vi "Input_Instrument_Positions.vi"(1 "Filepath to Save":path) -> (0 "Output string":string)   [LabVIEW 2010]
uses:
  Controls/ok_button.ctl
  Globals/Meas_global.vi
  Globals/Constants_global.vi
  Globals/Trav_pos_global.vi
panel:
  in  "OK":T1
  in  "Instrument positions when the traverse is at its origin":T2(array[cluster])=[{"Name"="", "X"=0.0, "Y"=0.0, "Z"=0.0, "Mounted On"=0}] {"Mounted On" items=["None", "No Traverse", "Tunnel3Traverse"]; "Z" format="%#.2f"; "Y" format="%#.2f"; "X" format="%#.2f"}
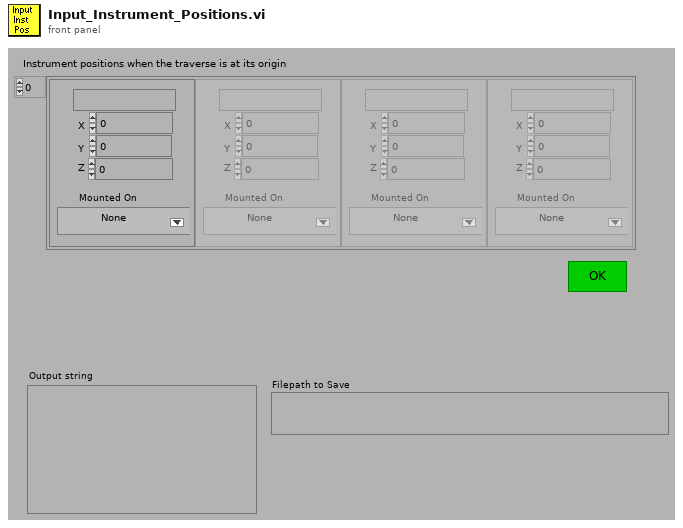
[diagram p1: front panel]
types:
  T1 = typedef "ok_button.ctl" = bool
  T2 = cluster{"Name":string, "X":dbl, "Y":dbl, "Z":dbl, "Mounted On":u16}[]
  T3 = cluster{"Name":string, "X":dbl, "Y":dbl, "Z":dbl}[]
  T4 = cluster{"Name":string, "X":dbl, "Y":dbl, "Z":dbl, "Mounted On":u16}
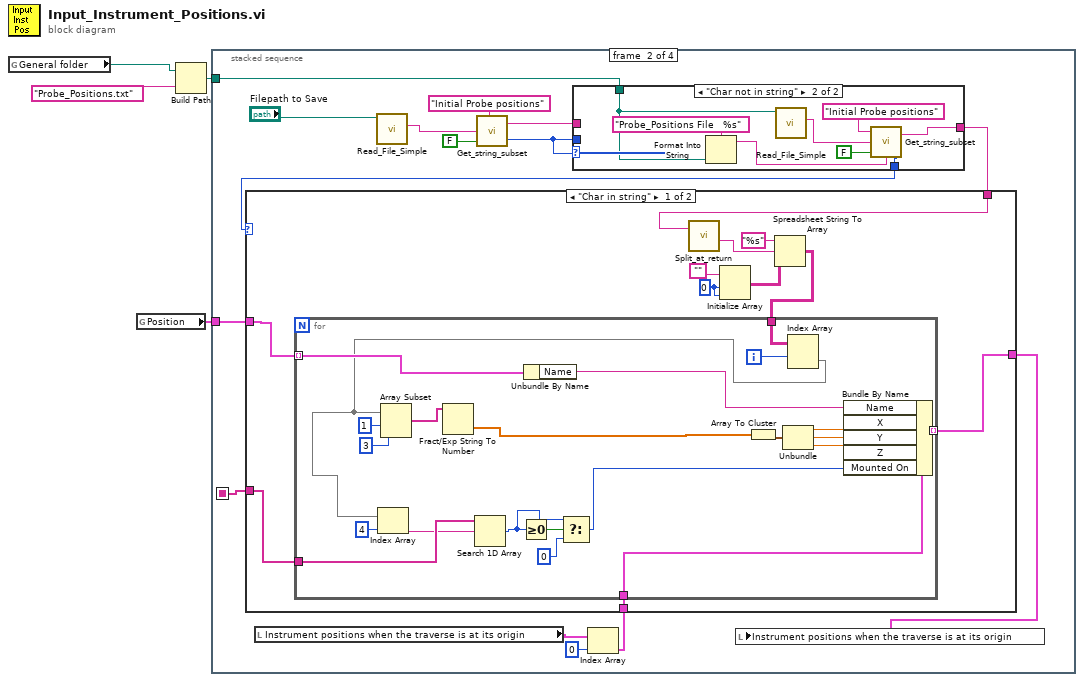
[diagram p0: block diagram]
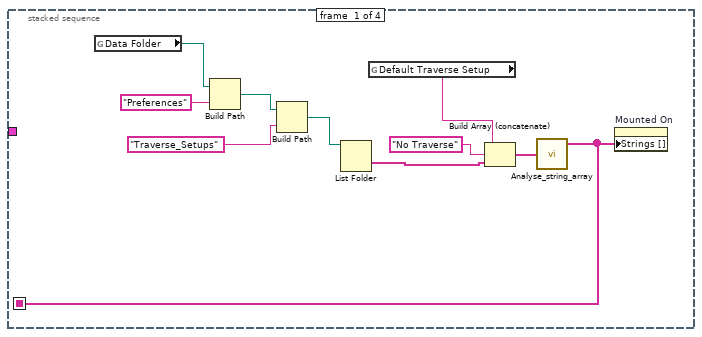
[diagram p2: hidden frame]
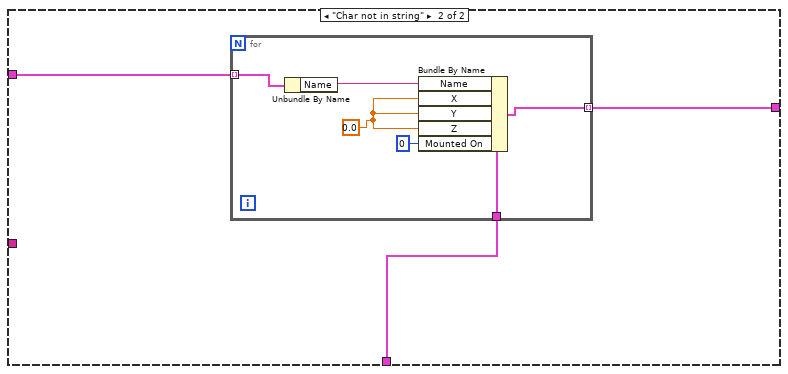
[diagram p4: hidden frame]
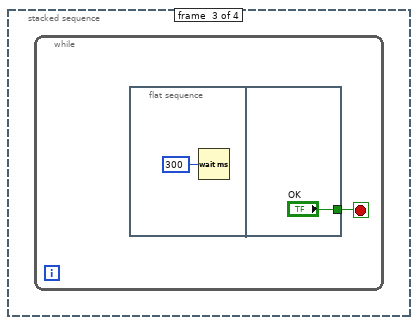
[diagram p5: hidden frame]
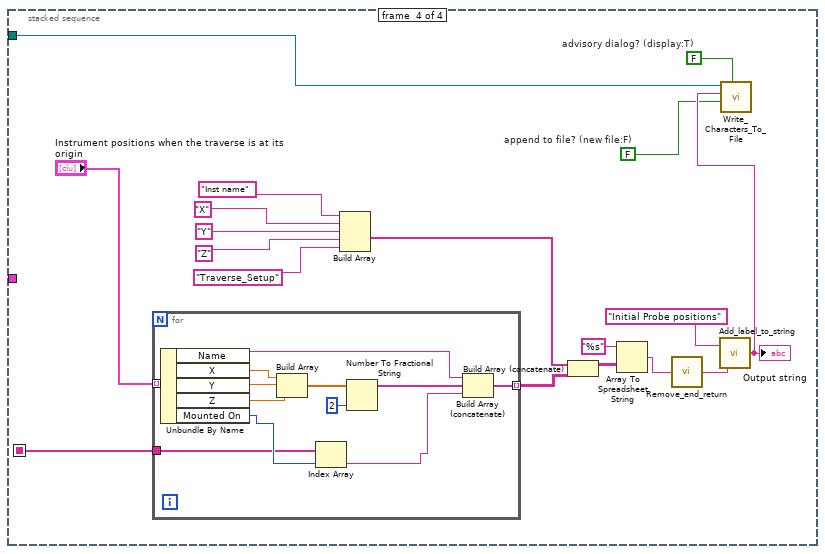
[diagram p6: hidden frame]
diagram:
  n1 = global read "Constants_global.vi" "General folder"() -> (w2:path)
  n2 = global read "Meas_global.vi" "Position"() -> (w4:T3)
  n3 = Build Path(base path=w2, name or relative path="Probe_Positions.txt") -> (appended path=w1:path)
  n4 = stacked-sequence {
    seq-local: [w5 _ _ _] -> [_ w23 _ w89]
    tunnel: w4 -> [_ w26 _ _]
    tunnel: w1 -> [_ w17 _ w85]
    frame #0 {
      n5 = global read "Constants_global.vi" "Data Folder"() -> (w11:path)
      n6 = Build Path(base path=w11, name or relative path="Preferences") -> (appended path=w13:path)
      n7 = Build Path(base path=w13, name or relative path="Traverse_Setups") -> (appended path=w10:path)
      n8 = List Folder(path=w10) -> (folder names=w7:string[])  [unwired: 1 in, 5 out]
      n9 = global read "Trav_pos_global.vi" "Default Traverse Setup"() -> (w9:string)
      n10 = Build Array (concatenate)(w9, "No Traverse" ("element"), w7) -> (w6:string[])
      n11 = call "Analyse_string_array.vi"("String array"=w6) -> ("Unique strings"=w5:string[])  [unwired: 2 out]
      n12 = property on="Mounted On" class="Ring (strict)"("Strings []"=w5) -> ()  [unwired: 2 in, 2 out]
    }
    frame #1 {
      n13 = local read "Instrument positions when the traverse is at its origin"() -> (w28:T2)
      n14 = call "Read_File_Simple.vi"("Filename"="Filepath to Save") -> ("string"=w20:string)  [unwired: 2 in, 7 out]
      n15 = call "Get_string_subset.vi"("Show Dialog?"=FALSE, "String to split"=w20, "File Label"="Initial Probe positions") -> ("Status"=w15:enum16{"Char in string", "Char not in string"}, "Output string"=w16:string)  [unwired: 1 in]
      n16 = case shown="\"Char not in string\"" w15 {
        tunnel: [w30 w36] -> w29
        tunnel: [w31 w35] -> w18
        tunnel: w17 -> [_ w33]
        tunnel: w16 -> [w31 _]
        tunnel: w15 -> [w30 _]
        frame "Char in string" {
        }
        frame "Char not in string" {
          n17 = Format Into String(format string="Probe_Positions File   %s", w33) -> (resulting string=w32:string)  [unwired: 2 in, 1 out]
          n18 = call "Read_File_Simple.vi"("Filename"=w33) -> ("string"=w37:string)  [unwired: 2 in, 7 out]
          n19 = call "Get_string_subset.vi"("String Name"=w32, "Show Dialog?"=FALSE, "String to split"=w37, "File Label"="Initial Probe positions") -> ("Status"=w36:enum16{"Char in string", "Char not in string"}, "Output string"=w35:string)
        }
      }
      n20 = Index Array(array=w28, index=0) -> (element=w25:T4)
      n21 = case shown="\"Char in string\"" w29 {
        tunnel: w26 -> [w41 w75]
        tunnel: w25 -> [w45 w74]
        tunnel: [w44 w73] -> w24
        tunnel: w23 -> [w43 _]
        tunnel: w18 -> [w42 _]
        frame "Char in string" {
          w47 = 0 ("Dimension Size")
          n22 = call "Split_at_return.vi"("String"=w42) -> ("after substring"=w50:string)  [unwired: 1 in, 3 out]
          n23 = Initialize Array("", w47, w47) -> (w46:string[][])
          n24 = Spreadsheet String To Array(format string="%s", spreadsheet string=w50, array type (2D Dbl)=w46) -> (array=w40:string[][])  [unwired: 1 out]
          n25 = for {
            tunnel: [w63] -> w44 mode=indexing
            tunnel: w45 -> [w62]
            tunnel: w43 -> [w61]
            tunnel: w41 -> [w54] mode=indexing
            tunnel: w40 -> [w53]
            i -> [w52]
            n26 = Unbundle By Name(w54) -> ("Name"=w55:string)
            n27 = Index Array(array=w53, index (row)=w52) -> (element=w51:string[])  [unwired: 1 in]
            n28 = Index Array(array=w51, index=4) -> (element=w60:string)
            n29 = Array Subset(array=w51, index=1, length=3) -> (w70:string[])
            n30 = Fract/Exp String To Number(string=w70) -> (number=w69:dbl[])  [unwired: 4 out]
            n31 = Search 1D Array(1D array=w61, element=w60) -> (index of element=w58:i32)  [unwired: 1 out]
            n32 = Greater Or Equal To 0?(x=w58) -> (x >= 0?=w59:bool)
            n33 = Select(t=w58, s=w59, f=0) -> (s? t:f=w56:i32)
            n34 = Array To Cluster(array=w69) -> (cluster=w68:cluster{"[0]":dbl, "[1]":dbl, "[2]":dbl})
            n35 = Unbundle(w68) -> ("[0]"=w67:dbl, "[1]"=w66:dbl, "[2]"=w65:dbl)
            n36 = Bundle By Name(cluster=w62, "Name"=w55, "X"=w67, "Y"=w66, "Z"=w65, "Mounted On"=w56) -> (w63:T4)
          }
        }
        frame "Char not in string" {
          n37 = for {
            tunnel: w75 -> [w78] mode=indexing
            tunnel: w74 -> [w77]
            tunnel: [w76] -> w73 mode=indexing
            w79 = 0.0 ("Z")
            n38 = Unbundle By Name(w78) -> ("Name"=w81:string)
            n39 = Bundle By Name(cluster=w77, "Name"=w81, "X"=w79, "Y"=w79, "Z"=w79, "Mounted On"=u16 0) -> (w76:T4)
          }
        }
      }
      n40 = local write "Instrument positions when the traverse is at its origin"(w24) -> ()
    }
    frame #2 {
      n41 = while {
        stop <- w82 stop-if-true
        n42 = flat-sequence {
          tunnel: ["OK"] -> w82
          frame #0 {
            n43 = Wait (ms)(milliseconds to wait=u32 300) -> ()  [unwired: 1 out]
          }
          frame #1 {
          }
        }
      }
    }
    frame #3 {
      w86 = FALSE  # append to file? (new file:F)
      w87 = FALSE  # advisory dialog? (display:T)
      n44 = for {
        tunnel: "Instrument positions when the traverse is at its origin" -> [w114] mode=indexing
        tunnel: [w106] -> w96 mode=indexing
        tunnel: w89 -> [w104]
        n45 = Unbundle By Name(w114) -> ("Name"=w108:string, "X"=w113:dbl, "Y"=w112:dbl, "Z"=w111:dbl, "Mounted On"=w105:u16)
        n46 = Build Array(w113, w112, w111) -> (w109:dbl[])
        n47 = Index Array(array=w104, index=w105) -> (element=w103:string)
        n48 = Number To Fractional String(number=w109, precision (6)=i16 2) -> (F-format string=w107:string[])  [unwired: 2 out]
        n49 = Build Array (concatenate)(w108, w107, w103) -> (w106:string[])
      }
      n50 = Build Array("Inst name", "X", "Y", "Z", "Traverse_Setup") -> (w97:string[])
      n51 = Build Array (concatenate)(w97, w96) -> (w99:string[][])
      n52 = Array To Spreadsheet String(array=w99, 3:"%s" ("format string")) -> (spreadsheet string=w101:string)  [unwired: 1 out]
      n53 = call "Remove_end_return.vi"("Input string"=w101) -> ("Output string"=w100:string)
      n54 = call "Add_label_to_string.vi"("String to write"=w100, "File Label"="Initial Probe positions") -> ("Output string"=w88:string)
      "Output string" <- w88
      n55 = call "Write_Characters_To_File.vi"("file path (dialog if empty)"=w85, "advisory dialog? (display:T)"=w87, "character string"=w88, "append to file? (new file:F)"=w86) -> ()  [unwired: 1 in, 4 out]
    }
  }
